vi "InitializeLDC501.vi"(5 "Serial Configuration":T1={"Baud Rate"=9600, "Parity"=0, "Data Bits"=8, "Stop Bits"=10, "Flow Control"=2} {"Flow Control" items=["None", "XON/XOFF", "RTS/CTS", "XON/XOFF & RTS/CTS", "DTR/DSR", "XON/XOFF & DTR/DSR"]; "Stop Bits" items=["1.0"=10, "1.5"=15, "2.0"=20]; "Data Bits" items=["7"=7, "8"=8]; "Parity" items=["None", "Odd", "Even", "Mark", "Space"]; "Baud Rate" items=["300"=300, "600"=600, "1200"=1200, "2400"=2400, "4800"=4800, "9600"=9600, "19200"=19200]}, 8 "error in (no error)":errorcluster, 10 "ID Query (True)":bool=TRUE, 11 "VISA resource name":refnum<visa-resource-name>) -> (0 "error out":errorcluster, 3 "VISA resource name out":refnum<visa-resource-name>)   [LabVIEW 2021]
panel:
  out "read buffer":string
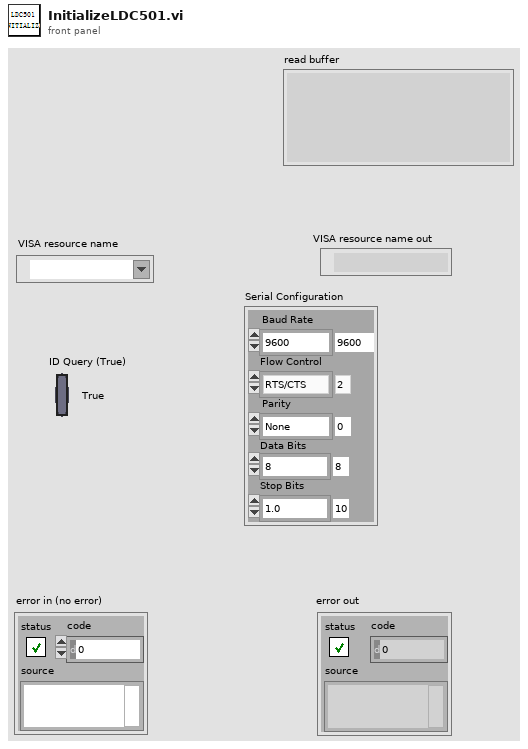
[diagram p1: front panel]
types:
  T1 = cluster{"Baud Rate":u32, "Parity":u16, "Data Bits":u16, "Stop Bits":u16, "Flow Control":u16}
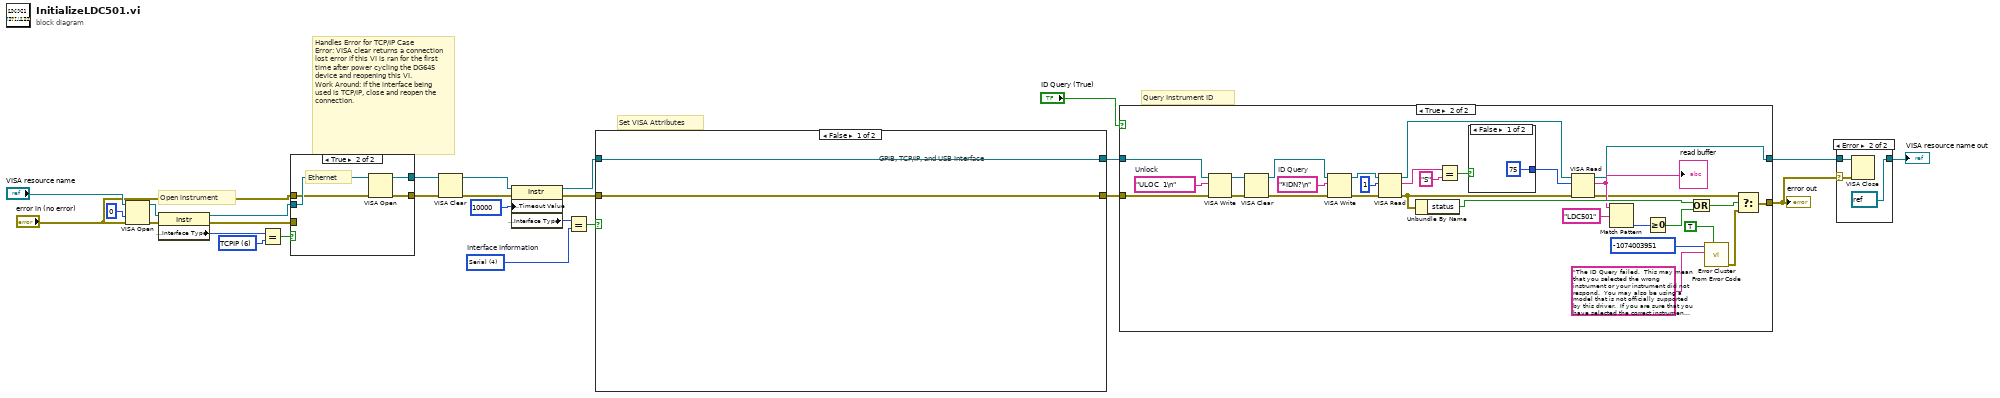
[diagram p0: block diagram]
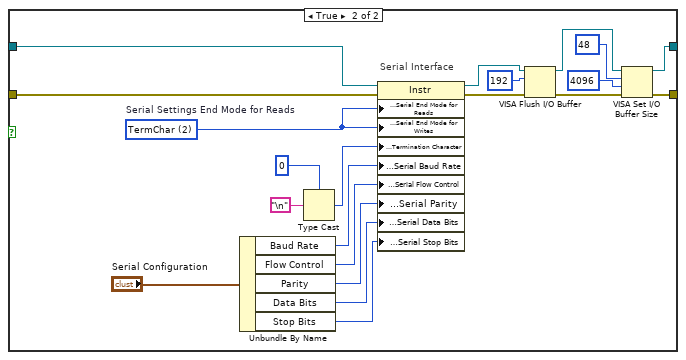
[diagram p4: hidden frame]
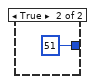
[diagram p6: hidden frame]
diagram:
  w13 = u16 6 items=["GPIB"=1, "VXI"=2, "GPIB-VXI"=3, "Serial"=4, "PXI"=5, "TCPIP"=6, "USB"=7] ("Interface Information:Interface Type")
  w20 = u16 4 items=["GPIB"=1, "VXI"=2, "GPIB-VXI"=3, "Serial"=4, "PXI"=5, "TCPIP"=6, "USB"=7]  # Interface Information
  # "Handles Error for TCP/IP Case\nError: VISA clear returns a connection lost error if this VI is ran for the first time after power cycling the DG645 device and reopening this VI.\nWork Around: If the interface being used is TCP/IP, close and reopen the connection."
  # "Set VISA Attributes"
  # "Query Instrument ID"
  # "Open instrument"
  n1 = VISA Open(access mode=u32 0, error in (no error)="error in (no error)", VISA resource name="VISA resource name") -> (VISA resource name=w15:refnum<visa-resource-name>, error out=w8:errorcluster)  [unwired: 2 in]
  n2 = property on="Property Node" class="Instr"(reference=w15, error in=w8) -> (reference out=w9:refnum<visa-resource-name>, error out=w11:errorcluster, "Interface Information:Interface Type"=w12:u16)
  n3 = Equal?(x=w12, y=w13) -> (x = y?=w14:bool)
  n4 = case shown="True" w14 {
    tunnel: [w27 w32] -> w16
    tunnel: w11 -> [w28 _]
    tunnel: w9 -> [w27 w31]
    tunnel: [w28 w29] -> w6
    tunnel: "error in (no error)" -> [_ w30]
    frame False {
      # "GPIB\nSerial"
    }
    frame True {
      # "Ethernet"
      n5 = VISA Open(error in (no error)=w30, VISA resource name=w31) -> (VISA resource name=w32:refnum<visa-resource-name>, error out=w29:errorcluster)  [unwired: 3 in]
    }
  }
  n6 = VISA Clear(VISA resource name=w16, error in (no error)=w6) -> (VISA resource name out=w17:refnum<visa-resource-name>, error out=w18:errorcluster)
  n7 = property on="Property Node" class="Instr"(reference=w17, error in=w18, "General Settings:Timeout Value"=u32 10000) -> (reference out=w22:refnum<visa-resource-name>, error out=w1:errorcluster, "Interface Information:Interface Type"=w25:u16)
  n8 = Equal?(x=w25, y=w20) -> (x = y?=w21:bool)
  n9 = case shown="False" w21 {
    tunnel: [w34 w53] -> w23
    tunnel: w22 -> [w34 w55]
    tunnel: [w33 w36] -> w2
    tunnel: w1 -> [w33 w35]
    frame False {
      # "GPIB, TCP/IP, and USB Interface"
    }
    frame True {
      w44 = u16 2 items=["None", "LastBit", "TermChar"]  # Serial Settings End Mode for Reads
      # "Serial Interface"
      n10 = Unbundle By Name("Serial Configuration") -> ("Baud Rate"=w42:u32, "Flow Control"=w38:u16, "Parity"=w40:u16, "Data Bits"=w41:u16, "Stop Bits"=w37:u16)
      n11 = Type Cast(type=u8 0, x="\n" ("Line Feed Constant")) -> (*(type *) &x=w43:u8)
      n12 = property on="Property Node" class="Instr"(reference=w55, error in=w35, "Serial Settings:Serial End Mode for Reads"=w44, "Serial Settings:Serial End Mode for Writes"=w44, "Message Based Settings:Termination Character"=w43, "Serial Settings:Serial Baud Rate"=w42, "Serial Settings:Serial Flow Control"=w38, "Serial Settings:Serial Parity"=w40, "Serial Settings:Serial Data Bits"=w41, "Serial Settings:Serial Stop Bits"=w37) -> (reference out=w50:refnum<visa-resource-name>, error out=w52:errorcluster)
      n13 = VISA Flush I/O Buffer(VISA resource name=w50, mask (16)=u16 192, error in (no error)=w52) -> (VISA resource name out=w54:refnum<visa-resource-name>, error out=w51:errorcluster)
      n14 = VISA Set I/O Buffer Size(VISA resource name=w54, mask (16)=u16 48, size (4096)=u32 4096 ("size (0)"), error in (no error)=w51) -> (VISA resource name out=w53:refnum<visa-resource-name>, error out=w36:errorcluster)
    }
  }
  n15 = case shown="True" "ID Query (True)" {
    tunnel: [w57 w60] -> w4
    tunnel: w23 -> [w57 w74]
    tunnel: [w56 w72] -> w3
    tunnel: w2 -> [w56 w71]
    frame False {
    }
    frame True {
      w75 = "ULOC  1\n"  # Unlock
      w84 = "*IDN?\n"  # ID Query
      n16 = VISA Write(VISA resource name=w74, write buffer=w75, error in (no error)=w71) -> (VISA resource name out=w68:refnum<visa-resource-name>, error out=w70:errorcluster)  [unwired: 1 out]
      n17 = VISA Clear(VISA resource name=w68, error in (no error)=w70) -> (VISA resource name out=w67:refnum<visa-resource-name>, error out=w69:errorcluster)
      n18 = VISA Write(VISA resource name=w67, write buffer=w84, error in (no error)=w69) -> (VISA resource name out=w87:refnum<visa-resource-name>, error out=w73:errorcluster)  [unwired: 1 out]
      n19 = VISA Read(VISA resource name=w87, byte count=u32 1, error in (no error)=w73) -> (VISA resource name out=w61:refnum<visa-resource-name>, read buffer=w66:string, error out=w59:errorcluster)  [unwired: 1 out]
      n20 = Unbundle By Name(w59) -> ("status"=w78:bool)
      n21 = Equal?(x=w66, y="S") -> (x = y?=w64:bool)
      n22 = case shown="False" w64 {
        tunnel: [u32 75 u32 51] -> w63
        frame False {
        }
        frame True {
        }
      }
      n23 = VISA Read(VISA resource name=w61, byte count=w63, error in (no error)=w59) -> (VISA resource name out=w60:refnum<visa-resource-name>, read buffer=w62:string, error out=w58:errorcluster)  [unwired: 1 out]
      "read buffer" <- w62
      n24 = Match Pattern(string=w62, regular expression="LDC501") -> (offset past match=w79:i32)  [unwired: 1 in, 3 out]
      n25 = Greater Or Equal To 0?(x=w79) -> (x >= 0?=w77:bool)
      n26 = Or(x=w78, y=w77) -> (x .or. y?=w76:bool)
      n27 = call <vilib>:"Error Cluster From Error Code.vi"("show call chain? (False)"=TRUE, "error message (\"\")"="The ID Query failed.  This may mean that you selected the wrong instrument or your instrument did not respond.  You may also be using a model that is not officially supported by this driver.  If you are sure that you have selected the correct instrument and it is responding, try disabling the ID Query." ("Source (VI Name)"), "error code (0)"=-1074003951 ("Code")) -> ("error out"=w83:errorcluster)  [unwired: 6 in]
      n28 = Select(t=w58, s=w76, f=w83) -> (s? t:f=w72:errorcluster)
    }
  }
  "error out" <- w3
  n29 = case shown="Error" w3 {
    selector: w3 -> [_ w91]
    tunnel: [w90 refnum<visa-resource-name> refnum ("VISA resource name out")] -> w5
    tunnel: w4 -> [w90 w92]
    frame No Error {
    }
    frame Error {
      n30 = VISA Close(VISA resource name=w92, error in (no error)=w91) -> ()  [unwired: 1 out]
    }
  }
  "VISA resource name out" <- w5
